vi "Lin_input.vi"() -> ()   [LabVIEW 2010]
panel:
  in  "stop":bool
  out "Waveform Graph":dynamicdata(graph)
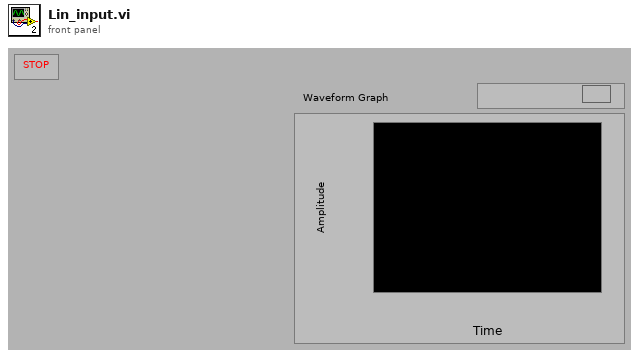
[diagram p1: front panel]
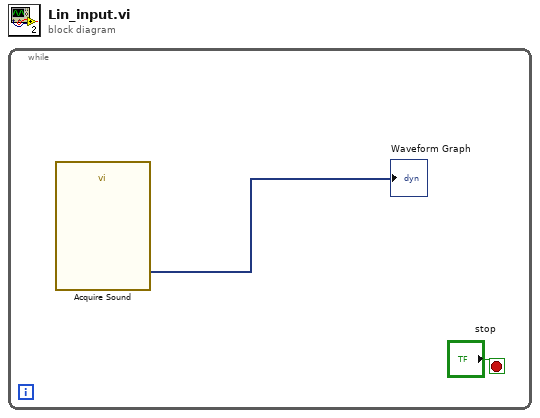
[diagram p0: block diagram]
diagram:
  n1 = while {
    stop <- "stop" stop-if-true
    n2 = call "Acquire Sound"() -> ("Data"=→"Waveform Graph":dynamicdata)  [unwired: 18 in, 1 out]
  }
